vi "Test Process Restart.vi"(8 "error in (no error)":errorcluster, 11 "Process Test In":refnum<class "Process Test.lvclass">) -> (0 "error out":errorcluster, 3 "Process Test Out":refnum<class "Process Test.lvclass">)   [LabVIEW 2020, in "Process Test.lvclass"]
uses:
  Process Test.lvclass
  C:/Program Files (x86)/National Instruments/LabVIEW 2020/vi.lib/Asteme/LUnit/Test Case.lvclass
  Framework/Process/Public/Lifecycle/Lifecycle State.ctl
  Mock Error Handler/Mock Error Handler.lvclass
  C:/Users/anton/Documents/GitHub/Triarc-Framework/source/Framework/Error Handler Interface/Error Handler Interface.lvclass
  Framework/Process/Process.lvclass/Process.ctl
  <vilib>/Asteme/LUnit/Test Case.lvclass/Test Case.ctl
  <vilib>/Asteme/LUnit/LUnit Assertion Result.lvclass/LUnit Assertion Result.ctl
  Framework/Process/Protected/Messaging/Enqueue Message.vi
  Framework/Process/Public/Lifecycle/Get Lifecycle State.vi
  Framework/Process/Private/SubVIs/Wait for finish.vi
  Framework/Process/Private/SubVIs/Set Lifecycle State.vi
  <vilib>/Asteme/LUnit/Palette/Pass If.vi
  <vilib>/Asteme/LUnit/Set Assertion Type.vi
  <vilib>/Asteme/LUnit/Palette/Pass.vi
  <vilib>/Asteme/LUnit/Palette/Fail.vi
  <vilib>/Utility/error.llb/Clear Errors.vi
  <vilib>/Asteme/LUnit/LUnit Write Assertion Type.vi
  <vilib>/Asteme/LUnit/Add test result.vi
  <vilib>/Asteme/LUnit/LUnit Write Passed.vi
  <vilib>/Asteme/LUnit/LUnit Get Test Case.vi
  <vilib>/Asteme/LUnit/Assertion Result/LUnit Get Test Name.vi
  <vilib>/Asteme/LUnit/LUnit Write Message.vi
  <vilib>/Asteme/LUnit/LUnit Write Description.vi
  <vilib>/Asteme/LUnit/Read Test Case Name.vi
  <vilib>/Utility/error.llb/Error Cluster From Error Code.vi
  <vilib>/Asteme/LUnit/LUnit Assertion Result.lvclass
  Framework/Process/Process.lvclass
  <vilib>/Asteme/LUnit/Test Case.lvclass
  C:/Users/anton/Documents/GitHub/Triarc-Framework/source/Framework Test/Base Class Test/Base Test.lvclass
  C:/Users/anton/Documents/GitHub/Triarc-Framework/source/Framework Test/Process Test/Process Test.lvclass
  C:/Users/anton/Documents/GitHub/Triarc-Framework/source/Framework/Base/Base.lvclass
  C:/Users/anton/Documents/GitHub/Triarc-Framework/source/Framework Test/Mock Error Handler/Mock Error Handler.lvclass
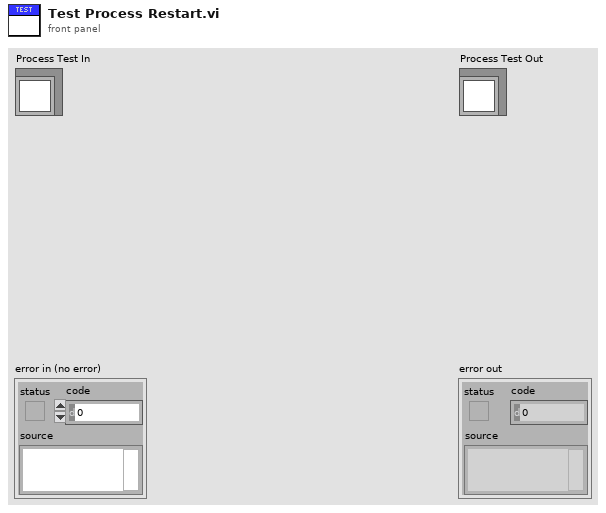
[diagram p1: front panel]
types:
  T1 = typedef "Process.lvclass/Lifecycle State.ctl" = enum16{"Uninitialized", "Initialized", "Started", "Running", "Stopped", "Finished"}
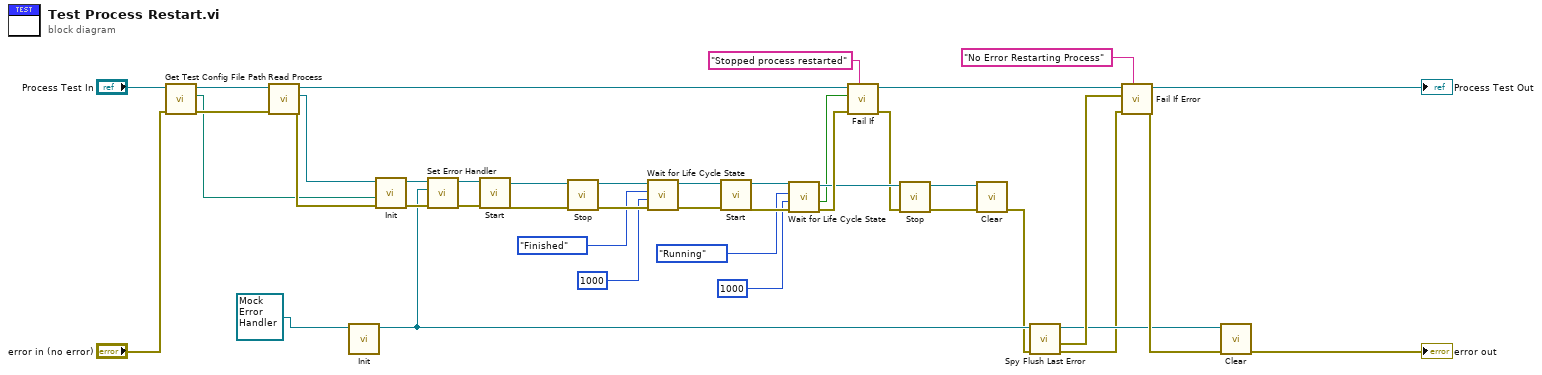
[diagram p0: block diagram]
diagram:
  n1 = call-dynamic "Get Test Config File Path.vi"("error in (no error)"="error in (no error)", "Base Class Test in"="Process Test In") -> ("error out"=w35:errorcluster, "Test config path"=w29:path, "Base Class Test out"=w38:refnum<class "Process Test.lvclass">)  [unwired: 7 in]
  n2 = call "Read Process.vi"("error in (no error)"=w35, "Process Test in"=w38) -> ("error out"=w36:errorcluster, "Process.lvclass"=w30:refnum<class "Process.lvclass">, "Process Test out"=w24:refnum<class "Process Test.lvclass">)  [unwired: 7 in]
  n3 = call-dynamic "Init.vi"("Mock Error Handler In"=refnum<class "Mock Error Handler.lvclass"> refnum ("Mock Error Handler.lvclass")) -> ("Mock Error Handler Out"=w8:refnum<class "Mock Error Handler.lvclass">)  [unwired: 9 in, 1 out]
  n4 = call-dynamic "Init.vi"("error in (no error)"=w36, "Config File Path"=w29, "Process In"=w30) -> ("error out"=w39:errorcluster, "Process Out"=w14:refnum<class "Process.lvclass">)  [unwired: 7 in]
  n5 = call "Set Error Handler.vi"("error in (no error)"=w39, "Error Handler"=w8, "Process In"=w14) -> ("error out"=w15:errorcluster, "Process Out"=w13:refnum<class "Process.lvclass">)  [unwired: 7 in]
  n6 = call "Start.vi"("error in (no error)"=w15, "Process In"=w13) -> ("error out"=w41:errorcluster, "Process Out"=w42:refnum<class "Process.lvclass">)  [unwired: 8 in]
  n7 = call "Stop.vi"("error in (no error)"=w41, "Process In"=w42) -> ("error out"=w31:errorcluster, "Process Out"=w27:refnum<class "Process.lvclass">)  [unwired: 7 in, 1 out]
  n8 = call "Wait for Life Cycle State.vi"("error in (no error)"=w31, "timeout in ms (-1)"=1000, "Lifecycle State"=Lifecycle_State."Finished", "Process In"=w27) -> ("error out"=w28:errorcluster, "Process Out"=w26:refnum<class "Process.lvclass">)  [unwired: 5 in, 1 out]
  n9 = call "Start.vi"("error in (no error)"=w28, "Process In"=w26) -> ("error out"=w34:errorcluster, "Process Out"=w21:refnum<class "Process.lvclass">)  [unwired: 8 in]
  n10 = call "Wait for Life Cycle State.vi"("error in (no error)"=w34, "timeout in ms (-1)"=1000, "Lifecycle State"=Lifecycle_State."Running", "Process In"=w21) -> ("error out"=w22:errorcluster, "timed out?"=w16:bool, "Process Out"=w20:refnum<class "Process.lvclass">)  [unwired: 5 in]
  n11 = call <vilib>:"Fail If.vi"("Description"="Stopped process restarted", "error in (no error)"=w22, "Fail?"=w16, "Test Case In"=w24) -> ("error out"=w17:errorcluster, "Test Case Out"=w11:refnum<class "Process Test.lvclass">)  [unwired: 6 in]
  n12 = call "Stop.vi"("error in (no error)"=w17, "Process In"=w20) -> ("error out"=w32:errorcluster, "Process Out"=w33:refnum<class "Process.lvclass">)  [unwired: 7 in, 1 out]
  n13 = call-dynamic "Clear.vi"("error in (no error)"=w32, "Process In"=w33) -> ("error out"=w4:errorcluster)  [unwired: 9 in]
  n14 = call "Spy Flush Last Error.vi"("error in (no error)"=w4, "Mock Error Handler In"=w8) -> ("error out"=w3:errorcluster, "Error"=w9:errorcluster, "Mock Error Handler Out"=w5:refnum<class "Mock Error Handler.lvclass">)  [unwired: 7 in]
  n15 = call <vilib>:"Fail If Error.vi"("Description"="No Error Restarting Process", "error in (no error)"=w3, "Assert error"=w9, "Test Case In"=w11) -> ("error out"=w7:errorcluster, "Test Case Out"=→"Process Test Out":refnum<class "Process Test.lvclass">)  [unwired: 6 in]
  n16 = call-dynamic "Clear.vi"("error in (no error)"=w7, "Mock Process In"=w5) -> ("error out"=→"error out":errorcluster)  [unwired: 9 in]
